vi "Check Records Done.vi"(8 "Increment?":bool, 9 "Records Finished":u16, 11 "Records to Acquire":u16) -> (1 "Updated Records Finished":u16, 2 "Is NumRecords >0?":bool, 3 "Records Done?":bool)   [LabVIEW 2012]
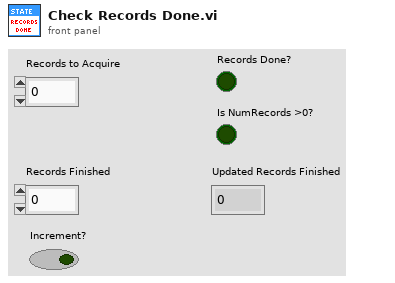
[diagram p1: front panel]
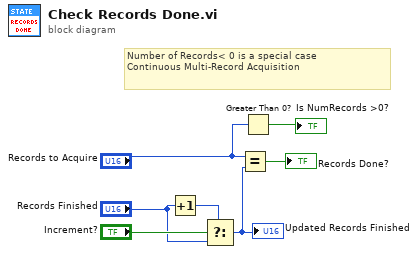
[diagram p0: block diagram]
diagram:
  # "Number of Records< 0 is a special case\nContinuous Multi-Record Acquisition"
  n1 = Increment(x="Records Finished") -> (x+1=w7:u16)
  n2 = Select(t=w7, s="Increment?", f="Records Finished") -> (s? t:f=w4:u16)
  "Updated Records Finished" <- w4
  n3 = Equal?(x="Records to Acquire", y=w4) -> (x = y?=→"Records Done?":bool)
  n4 = Greater Than 0?(x="Records to Acquire") -> (x > 0?=→"Is NumRecords >0?":bool)
